vi "Write to Device.vi"(8 "error in (no error)":errorcluster, 11 "Device in":refnum<class "PIC-Device.lvclass">) -> (0 "error out":errorcluster, 2 "Return":string[](array[string]), 3 "Device out":refnum<class "PIC-Device.lvclass">)   [LabVIEW 2020, in "PIC-Device.lvclass"]
doc: "Writes all to Device that is waiting in the \"Registers to write\" array of the class data.\nAfter an succesful write the \"Register to write\" array in the class data is emptied."
uses:
  PIC-Device.lvclass
  C:/Sandbox/RF Bench/Source Code/WiSpry Test Framework/Devices/Device.lvclass
  PIC-Device.lvclass/PIC-Device.ctl
  Controls/Register to Write.ctl
  Instruments/Power Supply/Power Supply.lvclass
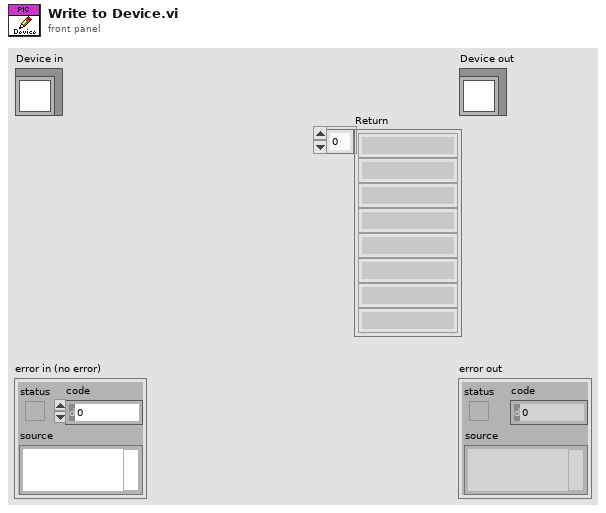
[diagram p1: front panel]
types:
  T1 = typedef "PIC-Device.lvclass/Register to Write.ctl" = cluster{"Register":u32, "Value":u32, "Dev Address":u32, "Physical Adress":u32}
  T2 = typedef "Device.lvclass/DC Offset Cluster.ctl" = cluster{"Enable":bool, "Use Array":bool, "Array":dbl[], "To From Cluster":cluster{"From":dbl, "To":dbl, "Step":dbl}, "Current Value":dbl, "DC Offset":refnum<class "Power Supply.lvclass">}
  T3 = enum16{"RFFE 2-wire", "WiSPI 3-wire spi_sel", "WiSPI 4-wire spi_sel", "ifxSPI 3-wire spi_sel", "WiSPI 3-wire dev add spi_sel"}
  T4 = cluster{"Register":bool, "Value":bool, "Dev Address":bool, "Physical Adress":bool}
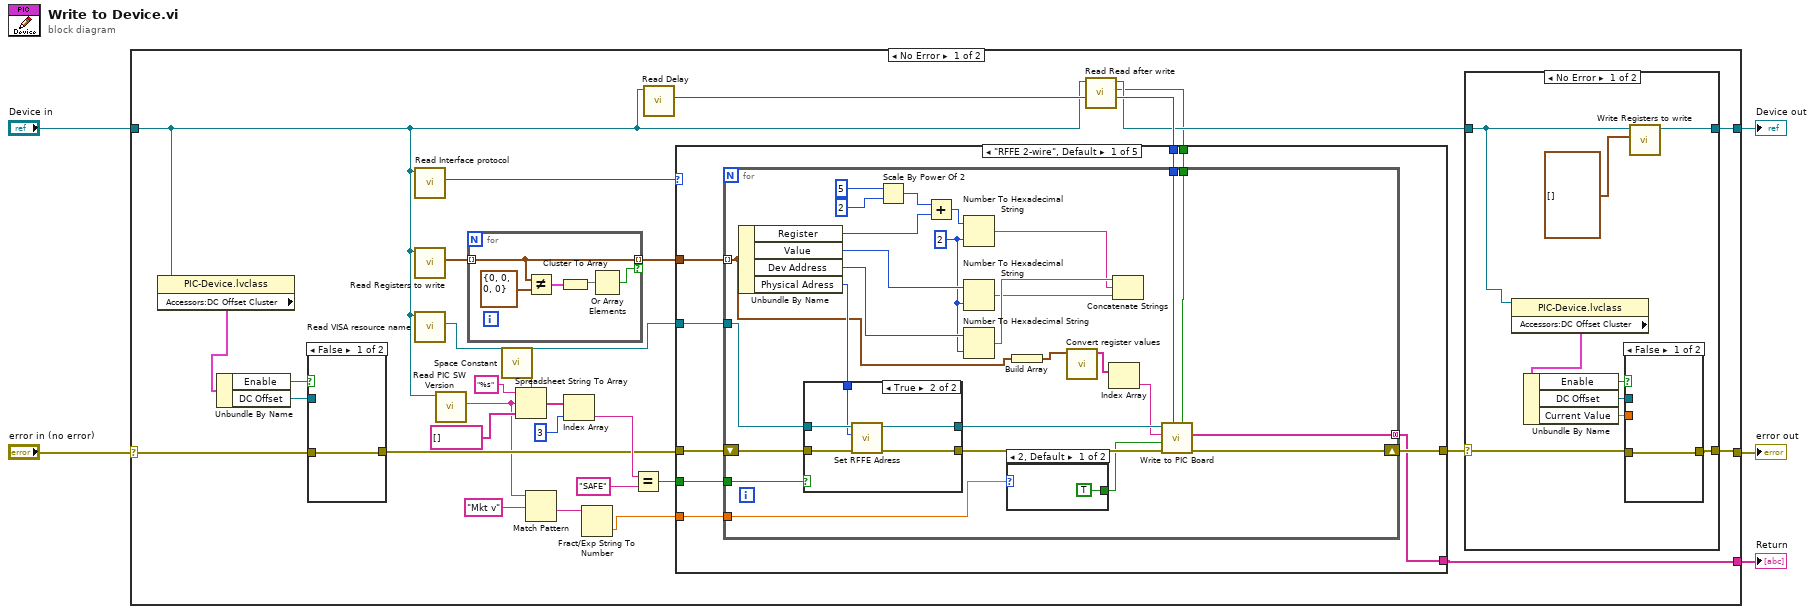
[diagram p0: block diagram]
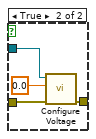
[diagram p2: hidden frame]
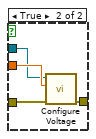
[diagram p3: hidden frame]
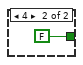
[diagram p5: hidden frame]
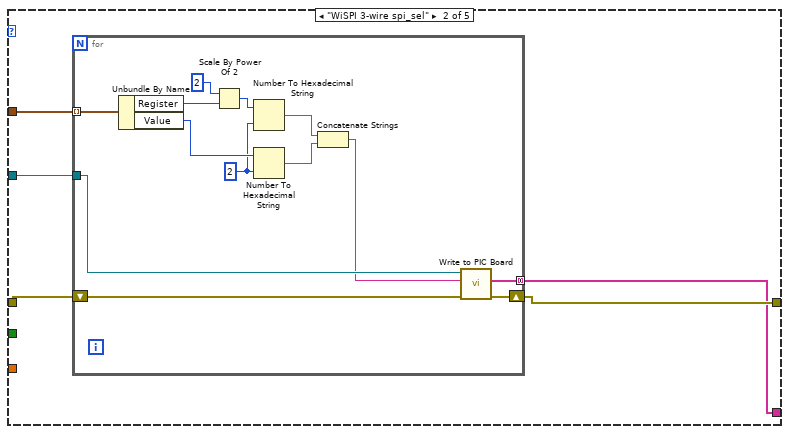
[diagram p7: hidden frame]
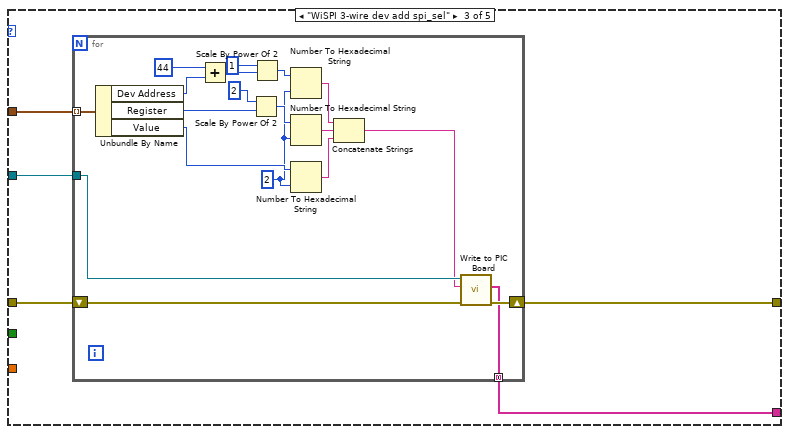
[diagram p8: hidden frame]
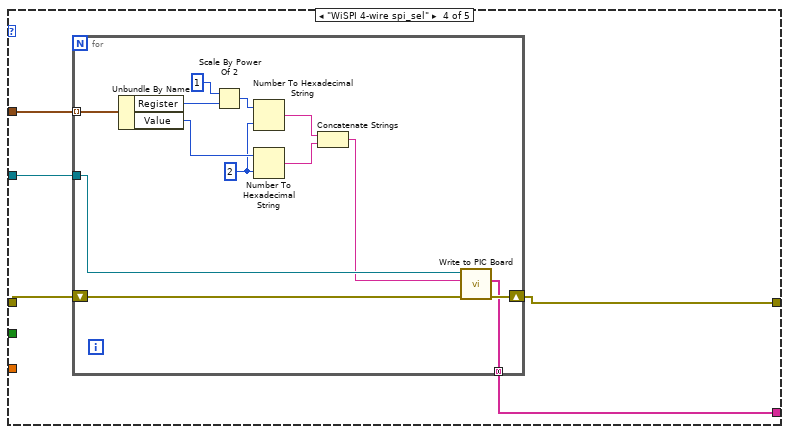
[diagram p9: hidden frame]
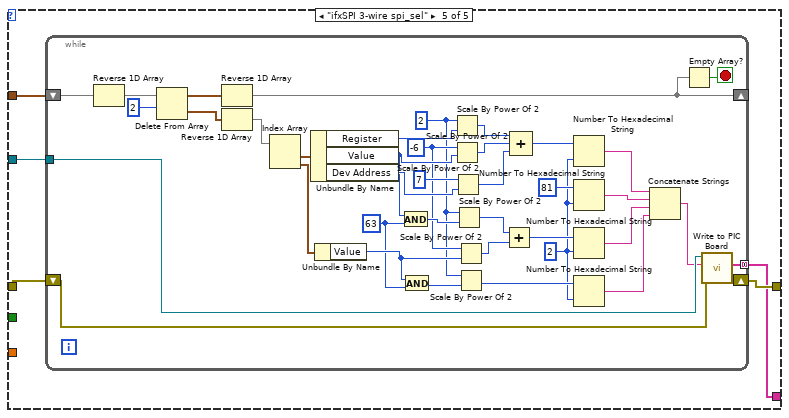
[diagram p10: hidden frame]
diagram:
  n1 = case shown="No Error" "error in (no error)" {
    selector: "error in (no error)" -> [w18 w211]
    tunnel: [w31 w211] -> w4
    tunnel: [w30 w210] -> w2
    tunnel: "Device in" -> [w8 w210]
    tunnel: [w15 _] -> w1
    frame No Error {
      n2 = property class="PIC-Device.lvclass"(reference=w8) -> ("Accessors:DC Offset Cluster"=w14:T2)  [unwired: 1 in, 2 out]
      n3 = Unbundle By Name(w14) -> ("Enable"=w19:bool, "DC Offset"=w17:refnum<class "Power Supply.lvclass">)
      n4 = case shown="False" w19 {
        tunnel: w18 -> [w35 w39]
        tunnel: w17 -> [_ w36]
        tunnel: [w35 w38] -> w16
        frame False {
        }
        frame True {
          n5 = call-dynamic "Configure Voltage.vi"("error in (no error)"=w39, "Voltage"=0.0, "Power Supply in"=w36) -> ("error out"=w38:errorcluster)  [unwired: 7 in, 1 out]
        }
      }
      n6 = call-dynamic "Read Interface protocol.vi"("Device in"=w8) -> ("Interface protocol"=w34:T3)  [unwired: 9 in, 1 out]
      n7 = call-dynamic "Read Registers to write.vi"("Device in"=w8) -> ("Registers to write"=w29:T1[])  [unwired: 9 in, 1 out]
      n8 = call-dynamic "Read VISA resource name.vi"("Device in"=w8) -> ("VISA resource name"=w33:refnum<visa-resource-name>)  [unwired: 9 in, 1 out]
      n9 = call "Read PIC SW Version.vi"("Device in"=w8) -> ("PIC SW Version"=w12:string)  [unwired: 9 in, 1 out]
      n10 = for {
        tunnel: w29 -> [w41] mode=indexing
        tunnel: [w41] -> w28 mode=indexing if=w40
        n11 = Not Equal?(x=w41, y=T1 {"Register"=0, "Value"=0, "Dev Address"=0, "Physical Adress"=0}) -> (x != y?=w43:T4)
        n12 = Cluster To Array(cluster=w43) -> (array=w42:bool[])
        n13 = Or Array Elements(Boolean array=w42) -> (logical OR=w40:bool)
      }
      n14 = call <vilib>:"Space Constant.vi"() -> ("String"=w26:string)
      n15 = Spreadsheet String To Array(delimiter (Tab)=w26, format string="%s", spreadsheet string=w12, array type (2D Dbl)=string[] []) -> (array=w24:string[])
      n16 = Match Pattern(string=w12, regular expression="Mkt v" ("format string")) -> (after substring=w11:string)  [unwired: 1 in, 3 out]
      n17 = Index Array(array=w24, index=3) -> (element=w22:string)
      n18 = Fract/Exp String To Number(string=w11) -> (number=w10:dbl)  [unwired: 3 in, 1 out]
      n19 = Equal?(x=w22, y="SAFE") -> (x = y?=w20:bool)
      n20 = call-dynamic "Read Delay.vi"("PIC-Device in"=w8) -> ("Delay"=w9:u32)  [unwired: 9 in, 1 out]
      n21 = call-dynamic "Read Read after write.vi"("Device in"=w8) -> ("Read after write"=w6:bool, "Device out"=w7:refnum<class "PIC-Device.lvclass">)  [unwired: 9 in]
      n22 = case shown="\"RFFE 2-wire\", Default" w34 {
        tunnel: w16 -> [w67 w110 w128 w152 w169]
        tunnel: w28 -> [w69 w109 w127 w151 w170]
        tunnel: w33 -> [w68 w108 w126 w150 w168]
        tunnel: [w66 w107 w125 w149 w167] -> w32
        tunnel: w20 -> [w65 _ _ _ _]
        tunnel: [w61 w106 w124 w148 w166] -> w15
        tunnel: w10 -> [w64 _ _ _ _]
        tunnel: w9 -> [w63 _ _ _ _]
        tunnel: w6 -> [w62 _ _ _ _]
        frame "RFFE 2-wire", Default {
          n23 = for {
            tunnel: w69 -> [w73] mode=indexing
            tunnel: w68 -> [w82]
            shift-right: [w84] -> w66
            shift-left: w67 -> [w96]
            tunnel: w65 -> [w79]
            tunnel: [w78] -> w61 mode=concatenating
            tunnel: w64 -> [w77]
            tunnel: w63 -> [w75]
            tunnel: w62 -> [w70]
            w88 = i16 2 ("width (-)")
            n24 = Unbundle By Name(w73) -> ("Register"=w92:u32, "Value"=w90:u32, "Dev Address"=w89:u32, "Physical Adress"=w80:u32)
            n25 = case shown="True" w79 {
              tunnel: w96 -> [w99 w105]
              tunnel: [w99 w104] -> w83
              tunnel: w82 -> [w100 w103]
              tunnel: [w100 w102] -> w81
              tunnel: w80 -> [_ w101]
              frame False {
              }
              frame True {
                n26 = call "Set RFFE Adress.vi"("error in (no error)"=w105, "Physical Adress"=w101, "VISA resource name"=w103) -> ("error out"=w104:errorcluster, "VISA resource name out"=w102:refnum<visa-resource-name>)  [unwired: 7 in]
              }
            }
            n27 = Scale By Power Of 2(n=u32 5, x=u32 2) -> (x*2^n=w93:u32)
            n28 = Add(x=w93, y=w92) -> (x+y=w91:u32)
            n29 = Number To Hexadecimal String(1:w88, 2:w91) -> (0:w86:string)
            n30 = Number To Hexadecimal String(1:w88, 2:w90) -> (0:w85:string)
            n31 = Number To Hexadecimal String(1:w88, 2:w89) -> (0:w87:string)
            n32 = case shown="2, Default" w77 {
              tunnel: [TRUE FALSE] -> w76
              frame 2, Default {
              }
              frame 4 {
              }
            }
            n33 = Build Array(w73) -> (w74:T1[])
            n34 = call "Convert register values.vi"("Register clusters"=w74) -> ("Register strings out"=w72:string[])  [unwired: 9 in, 1 out]
            n35 = Index Array(array=w72) -> (element=w71:string)  [unwired: 1 in]
            n36 = Concatenate Strings(w87, w86, w85) -> ()  [unwired: 1 out]
            n37 = call "Write to PIC Board.vi"("Read after write"=w70, "Delay between writes"=w75, "error in (no error)"=w83, "Ignore address in return"=w76, "String to write"=w71, "VISA Refnum in"=w81) -> ("Error Out"=w84:errorcluster, "Return"=w78:string[])  [unwired: 4 in]
          }
        }
        frame "WiSPI 3-wire spi_sel" {
          n38 = for {
            shift-right: [w112] -> w107
            shift-left: w110 -> [w115]
            tunnel: w109 -> [w123] mode=indexing
            tunnel: w108 -> [w114]
            tunnel: [w111] -> w106 mode=concatenating
            w118 = i16 2 ("width (-)")
            n39 = Unbundle By Name(w123) -> ("Register"=w121:u32, "Value"=w119:u32)
            n40 = Scale By Power Of 2(n=i16 2, x=w121) -> (x*2^n=w120:u32)
            n41 = Number To Hexadecimal String(1:w118, 2:w120) -> (0:w117:string)
            n42 = Number To Hexadecimal String(1:w118, 2:w119) -> (0:w116:string)
            n43 = Concatenate Strings(w117, w116) -> (w113:string)
            n44 = call "Write to PIC Board.vi"("error in (no error)"=w115, "String to write"=w113, "VISA Refnum in"=w114) -> ("Error Out"=w112:errorcluster, "Return"=w111:string[])  [unwired: 7 in]
          }
        }
        frame "WiSPI 3-wire dev add spi_sel" {
          n45 = for {
            shift-right: [w138] -> w125
            shift-left: w128 -> [w141]
            tunnel: w127 -> [w147] mode=indexing
            tunnel: w126 -> [w140]
            tunnel: [w129] -> w124 mode=concatenating
            w131 = i16 2 ("width (-)")
            n46 = Unbundle By Name(w147) -> ("Dev Address"=w137:u32, "Register"=w146:u32, "Value"=w144:u32)
            n47 = Add(x=u32 44, y=w137) -> (x+y=w134:u32)
            n48 = Scale By Power Of 2(n=i16 2, x=w146) -> (x*2^n=w145:u32)
            n49 = Scale By Power Of 2(n=i16 1, x=w134) -> (x*2^n=w132:u32)
            n50 = Number To Hexadecimal String(1:w131, 2:w132) -> (0:w130:string)
            n51 = Number To Hexadecimal String(1:w131, 2:w145) -> (0:w143:string)
            n52 = Number To Hexadecimal String(1:w131, 2:w144) -> (0:w142:string)
            n53 = Concatenate Strings(w130, w143, w142) -> (w139:string)
            n54 = call "Write to PIC Board.vi"("error in (no error)"=w141, "String to write"=w139, "VISA Refnum in"=w140) -> ("Error Out"=w138:errorcluster, "Return"=w129:string[])  [unwired: 7 in]
          }
        }
        frame "WiSPI 4-wire spi_sel" {
          n55 = for {
            shift-right: [w154] -> w149
            shift-left: w152 -> [w157]
            tunnel: w151 -> [w165] mode=indexing
            tunnel: w150 -> [w156]
            tunnel: [w153] -> w148 mode=concatenating
            w160 = i16 2 ("width (-)")
            n56 = Unbundle By Name(w165) -> ("Register"=w163:u32, "Value"=w161:u32)
            n57 = Scale By Power Of 2(n=i16 1, x=w163) -> (x*2^n=w162:u32)
            n58 = Number To Hexadecimal String(1:w160, 2:w162) -> (0:w159:string)
            n59 = Number To Hexadecimal String(1:w160, 2:w161) -> (0:w158:string)
            n60 = Concatenate Strings(w159, w158) -> (w155:string)
            n61 = call "Write to PIC Board.vi"("error in (no error)"=w157, "String to write"=w155, "VISA Refnum in"=w156) -> ("Error Out"=w154:errorcluster, "Return"=w153:string[])  [unwired: 7 in]
          }
        }
        frame "ifxSPI 3-wire spi_sel" {
          n62 = while {
            shift-right: [w205] -> _
            shift-left: w170 -> [w209]
            tunnel: w168 -> [w175]
            shift-right: [w172] -> w167
            shift-left: w169 -> [w174]
            tunnel: [w171] -> w166 mode=concatenating
            stop <- w204 stop-if-true
            w180 = i16 2 ("width (-)")
            w189 = u32 63 ("y")
            w191 = i16 -6 ("n")
            w183 = i16 2 ("n")
            n63 = Reverse 1D Array(array=w209) -> (reversed array=w208:T1[])
            n64 = Delete From Array(array=w208, length=2) -> (deleted portion=w203:T1[], array with subset deleted=w206:T1[])  [unwired: 1 in]
            n65 = Reverse 1D Array(array=w206) -> (reversed array=w205:T1[])
            n66 = Reverse 1D Array(array=w203) -> (reversed array=w202:T1[])
            n67 = Index Array(array=w202) -> (element #1=w201:T1, element #2=w200:T1)  [unwired: 2 in]
            n68 = Unbundle By Name(w201) -> ("Register"=w199:u32, "Value"=w193:u32, "Dev Address"=w198:u32)
            n69 = Unbundle By Name(w200) -> ("Value"=w190:u32)
            n70 = And(x=w193, y=w189) -> (x .and. y?=w192:u32)
            n71 = And(x=w190, y=w189) -> (x .and. y?=w182:u32)
            n72 = Scale By Power Of 2(n=w183, x=w199) -> (x*2^n=w197:u32)
            n73 = Scale By Power Of 2(n=w191, x=w193) -> (x*2^n=w196:u32)
            n74 = Scale By Power Of 2(n=i16 7, x=w198) -> (x*2^n=w195:u32)
            n75 = Scale By Power Of 2(n=w183, x=w192) -> (x*2^n=w188:u32)
            n76 = Scale By Power Of 2(n=w191, x=w190) -> (x*2^n=w184:u32)
            n77 = Scale By Power Of 2(n=w183, x=w182) -> (x*2^n=w181:u32)
            n78 = Add(x=w188, y=w184) -> (x+y=w185:u32)
            n79 = Compound Arithmetic op=ADD(w197, w196, w195) -> (w187:u32)
            n80 = Number To Hexadecimal String(1:w180, 2:w187) -> (0:w179:string)
            n81 = Number To Hexadecimal String(1:w180, 2:81 ("number")) -> (0:w178:string)
            n82 = Number To Hexadecimal String(1:w180, 2:w185) -> (0:w177:string)
            n83 = Number To Hexadecimal String(1:w180, 2:w181) -> (0:w176:string)
            n84 = Concatenate Strings(w179, w178, w177, w176) -> (w173:string)
            n85 = Empty Array?(array=w205) -> (empty?=w204:bool)
            n86 = call "Write to PIC Board.vi"("error in (no error)"=w174, "String to write"=w173, "VISA Refnum in"=w175) -> ("Error Out"=w172:errorcluster, "Return"=w171:string[])  [unwired: 7 in]
          }
        }
      }
      n87 = case shown="No Error" w32 {
        selector: w32 -> [w49 w59]
        tunnel: [w48 w59] -> w31
        tunnel: w7 -> [w46 w60]
        tunnel: [w53 w60] -> w30
        frame No Error {
          n88 = property class="PIC-Device.lvclass"(reference=w46) -> ("Accessors:DC Offset Cluster"=w45:T2)  [unwired: 1 in, 2 out]
          n89 = Unbundle By Name(w45) -> ("Enable"=w50:bool, "DC Offset"=w51:refnum<class "Power Supply.lvclass">, "Current Value"=w47:dbl)
          n90 = case shown="False" w50 {
            tunnel: w49 -> [w54 w58]
            tunnel: w51 -> [_ w55]
            tunnel: [w54 w57] -> w48
            tunnel: w47 -> [_ w56]
            frame False {
            }
            frame True {
              n91 = call-dynamic "Configure Voltage.vi"("error in (no error)"=w58, "Voltage"=w56, "Power Supply in"=w55) -> ("error out"=w57:errorcluster)  [unwired: 7 in, 1 out]
            }
          }
          n92 = call-dynamic "Write Registers to write.vi"("Registers to write"=T1[] [], "Device in"=w46) -> ("Device out"=w53:refnum<class "PIC-Device.lvclass">)  [unwired: 9 in]
        }
        frame Error {
        }
      }
    }
    frame Error {
    }
  }
  "error out" <- w4
  "Device out" <- w2
  "Return" <- w1
